vi "Close.vi"(8 "error in":errorcluster, 11 "KinectSensor References":T1) -> (0 "error out":errorcluster)   [LabVIEW 2014, in "LVH-KinectOne.lvlib"]
doc: "Closes the current Kinect session."
uses:
  LVH-KinectOne.lvlib
  Private/Type Defs/KinectSensor References.ctl
  Microsoft.Kinect
  C:/github/labviewhacker/LVH-KinectOne/LabVIEW/vi.lib/LabVIEW Hacker/KinectOne/Private/Libs/BodyFrameDataInterface.dll
  Private/Libs/BodyFrameDataInterface.dll
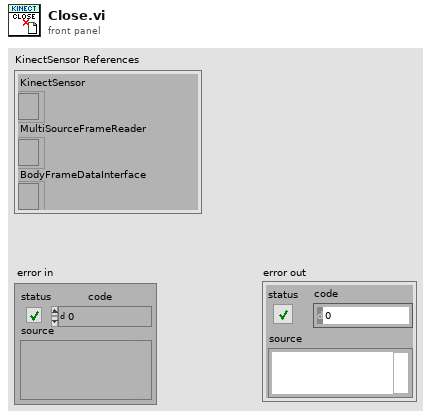
[diagram p1: front panel]
types:
  T1 = typedef "LVH-KinectOne.lvlib/KinectSensor References.ctl" = cluster{"KinectSensor":refnum<k24>, "MultiSourceFrameReader":refnum<k24>, "BodyFrameDataInterface":refnum<k24>}
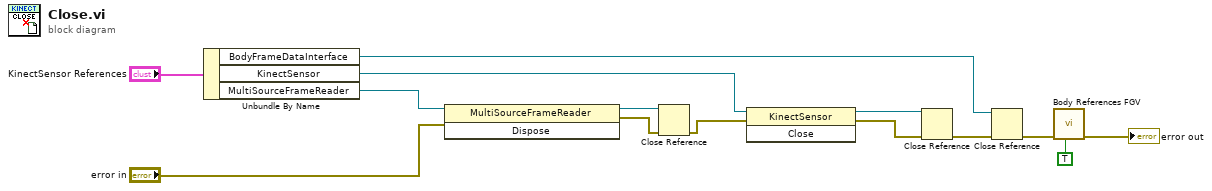
[diagram p0: block diagram]
diagram:
  n1 = Unbundle By Name("KinectSensor References") -> ("BodyFrameDataInterface"=w4:refnum<k24>, "KinectSensor"=w6:refnum<k24>, "MultiSourceFrameReader"=w7:refnum<k24>)
  n2 = invoke class="MultiSourceFrameReader" method="Dispose"(reference=w7, error in="error in") -> (reference out=w14:refnum<k24>, error out=w13:errorcluster)  [unwired: 1 in, 1 out]
  n3 = Close Reference(reference=w14, error in (no error)=w13) -> (error out=w12:errorcluster)
  n4 = invoke class="KinectSensor" method="Close"(reference=w6, error in=w12) -> (reference out=w11:refnum<k24>, error out=w10:errorcluster)  [unwired: 1 in, 1 out]
  n5 = Close Reference(reference=w11, error in (no error)=w10) -> (error out=w5:errorcluster)
  n6 = Close Reference(reference=w4, error in (no error)=w5) -> (error out=w3:errorcluster)
  n7 = call "Body References FGV.vi"("Destroy References?"=TRUE, "error in (no error)"=w3) -> ("error out"=→"error out":errorcluster)  [unwired: 9 in]
